vi "Machine Info.vi"() -> (0 "Type":string, 1 "Serial Number":string, 2 "Primary IP":string, 3 "Machine ID":string)   [LabVIEW 2020, in "Volatus.lvlib" / "Volatus Core.lvclass"]
uses:
  Volatus Core.lvclass
  Volatus Core.lvclass/Volatus Core.ctl
  <resource>/objmgr/nisysapi.rc
  <vilib>/nisyscfg/nisyscfg.lvlib
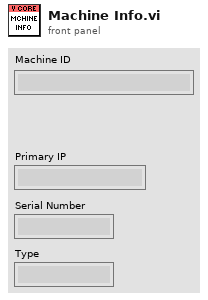
[diagram p1: front panel]
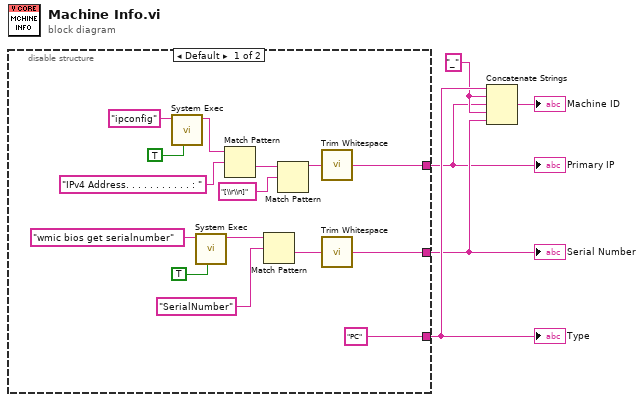
[diagram p0: block diagram]
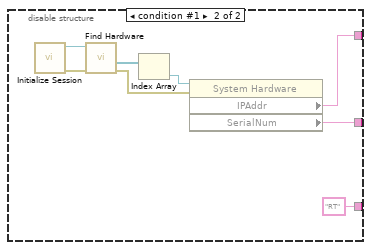
[diagram p2: hidden frame]
diagram:
  w4 = "_"
  n1 = disable-structure shown="Default" {
    disable-tunnel: [w14 w27] -> w2
    disable-tunnel: [w9 w26] -> w3
    disable-tunnel: ["PC" "RT"] -> w5
    frame condition #0 (active) {
      n2 = call <vilib>:"System Exec.vi"("run minimized? (F)"=TRUE, "command line"="ipconfig") -> ("standard output"=w19:string)  [unwired: 6 in, 3 out]
      n3 = call <vilib>:"System Exec.vi"("run minimized? (F)"=TRUE, "command line"="wmic bios get serialnumber") -> ("standard output"=w12:string)  [unwired: 6 in, 3 out]
      n4 = Match Pattern(string=w19, regular expression="IPv4 Address. . . . . . . . . . . : ") -> (after substring=w17:string)  [unwired: 1 in, 3 out]
      n5 = Match Pattern(string=w12, regular expression="SerialNumber") -> (after substring=w10:string)  [unwired: 1 in, 3 out]
      n6 = Match Pattern(string=w17, regular expression="[\\r\\n]") -> (before substring=w15:string)  [unwired: 1 in, 3 out]
      n7 = call <vilib>:"Trim Whitespace.vi"("string"=w15) -> ("trimmed string"=w14:string)  [unwired: 1 in]
      n8 = call <vilib>:"Trim Whitespace.vi"("string"=w10) -> ("trimmed string"=w9:string)  [unwired: 1 in]
    }
    frame condition #1 {
      n9 = call <vilib>:"Initialize Session.vi"() -> ("error out"=w22:errorcluster, "Session out"=w25:refnum<k21>)  [unwired: 10 in]
      n10 = call <vilib>:"Find Hardware.vi"("error in (no error)"=w22, "Session in"=w25) -> ("error out"=w21:errorcluster, "Resources out"=w24:refnum<k20>[])  [unwired: 6 in, 2 out]
      n11 = Index Array(array=w24) -> (element=w23:refnum<k20>)  [unwired: 1 in]
      n12 = property class="System Hardware"(reference=w23, error in=w21) -> ("IPAddr"=w27:string, "SerialNum"=w26:string)  [unwired: 2 out]
    }
  }
  "Primary IP" <- w2
  "Serial Number" <- w3
  "Type" <- w5
  n13 = Concatenate Strings(w5, w4, w2, w4, w3) -> (→"Machine ID":string)
